vi "AlliGator Phasor Algebra Calculator.vi"(7 "XYGraph in":T7, 8 "error in (no error)":errorcluster, 9 "Phasor Plot Destination":T1, 10 "Phasor Plot Algebra Output":T2 {"1-Exp Lifetime" min=0.0; "Delay" min=0.0}, 11 "Data Value Reference in":refnum<data-value>) -> (0 "error out":errorcluster, 1 "Message":string, 3 "Data Value Reference out":refnum<data-value>)   [LabVIEW 2021, in "AlliGator Phasor Graph.lvlib"]
doc: "Implements user-requested calculations on phsor plots."
uses:
  AlliGator Phasor Graph.lvlib
  AlliGator Internal Variables v2.ctl
  <vilib>/vision/Image Controls.llb/IMAQ Image.ctl
  AlliGator Gate Image Set.ctl
  AlliGator FLI Dataset Type.ctl
  AlliGator Data Series Type.ctl
  AlliGator Dataset Channel.ctl
  AlliGator Gate Arithmetic.ctl
  AlliGator Displayed Image.ctl
  Image/Named ROI Description.ctl
  AlliGator Decay Metadata v3.ctl
  AlliGator Decay Background Subtraction Info.ctl
  AlliGator Baseline Subtraction Method.ctl
  Graphs/XY Graph/XY Graph Plot Shift Parameters.ctl
  Graphs/XY Graph/XY Graph Plot Shift Method.ctl
  AlliGator Decay Extrapolation Parameters.ctl
  Phasor/Calibration Phasor (m, phi).ctl
  Phasor/Phasor Reference Series.ctl
  Phasor/Phasor Calibration Map v2.ctl
  Phasor/Phasor (g, s).ctl
  AlliGator Raw Phasor Plot Data v4.ctl
  Phasor/Phasor Standard Deviation Options.ctl
  AlliGator Phasor Multi-Harmonic Data.ctl
  Phasor/Phasor Harmonic Data.ctl
  AlliGator Decay Fit Options & Parameters v2.ctl
  Fits/IRF(X)PSED/Decay Fit Options v2.ctl
  Fits/Decay Convolution/Decay Model.ctl
  Fits/Residual Type.ctl
  Fits/IRF(X)PSED/Fit Weights Type.ctl
  Fits/Non-linear Fitting Method v2.ctl
  Fits/Fit Calculation Method.ctl
  Fits/Non-linear Fitting Algorithm.ctl
  AlliGator Decay Fit Parameter Constraints 2.ctl
  Fits/IRF(X)PSED/Decay Fit Parameters In List.ctl
  Fits/IRF(X)PSED/MLE Baseline Offset Type.ctl
  AlliGator Decay Preprocessing Parameters.ctl
  Fits/IRF(X)PSED/Decay Fit Parameters & Derived Quantities List.ctl
  Graphs/XY Graph/XY Graph Refnum.ctl
  AlliGator 2-Phasor Plot Multiplication.ctl
  Phasor/Phasor Operation.ctl
  Phasor/Phasor (m, phi).ctl
  Phasor/Phasor Representation.ctl
  AlliGator Phasor Plot Destination.ctl
  Graphs/Plot Point Style.ctl
  Graphs/LabVIEW Plot Interpolation.ctl
  02880097-ea6c-4998-a11e-0251a8662878.vi
  <vilib>/Utility/error.llb/Error Cluster From Error Code.vi
  Math/ix/ix (DBL).vi
  Graphs/XY Graph/XY Graph Add Single Plot with Name.vi
  <vilib>/ErrorRing/Error Ring.xnode
  Graphs/XY Graph/XY Graph Add-Ons.lvlib
  AlliGator Settings.lvlib
  Math/Math.lvlib
  Phasor/Phasor.lvlib
  Graphs/Graphs.lvlib
  Image/Image.lvlib
  AlliGator Decay Preprocessing.lvlib
  AlliGator Files.lvlib
  AlliGator Phasor Plot.lvlib
  AlliGator Source Image.lvlib
  Fits/Fits.lvlib
  AlliGator Decay Fit.lvlib
  AlliGator Decay Fit Parameter Map.lvlib
  AlliGator Internal Variables.lvlib
  AlliGator Dual-Channel Datasets.lvlib
panel:
  # "see the AlliGator License on the block diagram (Ctrl+E or Window:Show Block Diagram)"
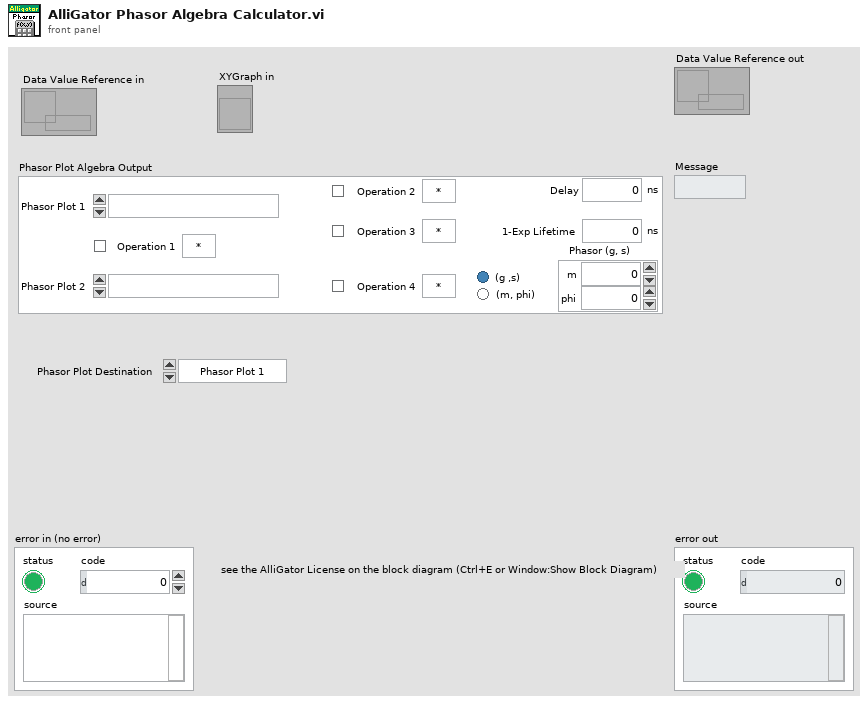
[diagram p1: front panel]
types:
  T1 = typedef "AlliGator Phasor Graph.lvlib/AlliGator Phasor Plot Destination.ctl" = enum32{"Phasor Plot 1", "Phasor Plot 2", "New Phasor Plot"}
  T2 = typedef "AlliGator Phasor Graph.lvlib/AlliGator 2-Phasor Plot Multiplication.ctl" = cluster{"Phasor Plot 1":u16, "Operation 1":T3, "Phasor Plot 2":u16, "Operation 2":T3, "Delay":dbl[unit], "Operation 3":T3, "1-Exp Lifetime":dbl[unit], "Operation 4":T3, "Phasor (g, s)":T4, "Phasor (m, phi)":T5, "Phasor Representation":T6, "Use Operation 1":bool, "Use Operation 2":bool, "Use Operation 3":bool, "Use Operation 4":bool}
  T3 = typedef "Phasor.lvlib/Phasor Operation.ctl" = enum16{"*", "/"}
  T4 = typedef "Phasor.lvlib/Phasor (g, s).ctl" = cluster{"g":dbl, "s":dbl}
  T5 = typedef "Phasor.lvlib/Phasor (m, phi).ctl" = cluster{"m":dbl, "phi":dbl}
  T6 = typedef "Phasor.lvlib/Phasor Representation.ctl" = enum32{"(g, s)", "(m, phi)"}
  T7 = typedef "XY Graph Add-Ons.lvlib/XY Graph Refnum.ctl" = refnum<vi>
  T8 = typedef "Graphs.lvlib/Plot Point Style.ctl" = enum16{"not defined", "None", "Empty Circle", "Filled Circle", "Thick Circle", "Dotted Circle", "Empty Square", "Filled Square", "Thick Square", "Dotted Square", "Small Filled Square", "Dot", "Cross", "Tiny Cross", "Large X", "Small x", "Diamond", "Small Empty Square"}
  T9 = typedef "AlliGator Internal Variables.lvlib/AlliGator Internal Variables v2.ctl" = cluster{"Displayed Image":T10, "White Light Image":T10, "Mask Image":T10, "ROI Mask Image":T10, "Current Dataset Images 1":T11, "Background Dataset Images 1":T11, "Current Dataset Images 2":T11, "Background Dataset Images 2":T11, "Current Dataset Arithmetic Images":T11, "Accumulated Dataset Images 1":T11, "Accumulated Dataset Images 2":T11, "Accumulated Dataset Arithmetic Images":T11, "Phasor Plot Image":T10, "Decay Fit Parameter Map Image":T10, "Single Data Point Path":path, "White Light Image Path":path, "Mask Image Path":path, "Time-Series Folder":path, "[Time-Series Paths]":path[], "Current Dataset":i32, "Single Dataset Type":T12, "Current Folder":string, "AlliGator Data Series Type":T13, "# Datasets":i32, "Dual-Channel Dataset":bool, "Selected Channel Name":string, "Dataset Channel":T14, "Channel Arithmetic":T15, "Dual-Channel Background Dataset":bool, "Background Channel":T14, "Dual-Channel Accumulated Dataset":bool, "Start Time":dbl, "[Time-Series Timestamps]":dbl[], "[Intensity Corrections]":dbl[], "Time Series Script":bool, "Type of Displayed Image":T16, "Gate Image Slide":u16, "# Gates":i32, "ROIs":T17[], "ROI Decay":cluster{"t Array":dbl[], "I Array":dbl[]}, "Valid Decay":bool, "Decay  Metadata":T19, "Reference Decay Plot Name":string, "Reference Decay":cluster{"t Array":dbl[], "I Array":dbl[]}, "Decay Shift Plot":cluster{"Time Stamps":dbl[], "Decay Shifts":dbl[]}, "[Decays Max Values]":sgl[], "[Decays Min Values]":sgl[], "Calibration Phasor":T25, "Calibration Phasor Series":T26, "Phasor Calibration Map":T27, "Calibration Map MD5 Digest":string, "Last Raw Phasor":T4, "Last Calibrated Phasor":T4, "Last Calibrated Phasor SDV":T4, "Phasor Graph:Phasor Plot":cluster{"g Array":dbl[], "s Array":dbl[]}, "Phasor Graph:Phasor SDV Plot":cluster{"g Array":dbl[], "s Array":dbl[]}, "[Phasor Graph:Raw Phasor Plots]":T28[], "Phasor Plot locked to Ref 1":i32, "[Phasor Plot(s) locked to Ref 1]":i32[], "[Phasor Plot(s) locked to Ref 2]":i32[], "[Pixel Phasors]":T4[], "[[Sum Image]]":dbl[][], "[[CSG Phasors]]":csg[][], "[[Valid Pixel?]]":bool[][], "I/m/phi Dataset":cluster{"I/m/phi Dataset?":bool, "Base Frequency":dbl[unit], "Harmonic Orders":u8[]}, "Multi Phasor Plot Data":T30, "Decay Fit Options & Parameters":T32, "Fit Options: Decay Preprocessing Parameters":T43, "Fit Options: Reference Decay":cluster{"t Array":dbl[], "I Array":dbl[]}, "Is Full Image Parameters Map":bool, "Is Single-Pixels Parameters Map":bool, "NLSF Parameters Map X Resolution":i32, "NLSF Parameters Map Y Resolution":i32, "[Single Decay Fit Parameters]":dbl[], "Fit Model":T34, "[[Multiple Decays Fit Parameters]]":dbl[][], "[[Multiple Decays Fit Parameter SDVs]]":dbl[][], "[[IRFs]]":dbl[][], "IRF Array Time Axis":dbl[], "Decay Array Time Axis":dbl[], "[Decay Fit Parameter Names]":T44[], "[[Phasor Ratios]]":dbl[][], "[[Average Lifetimes]]":dbl[][], "Amplitude Weighted Average Lifetime":bool, "[Decay Sum]":dbl[], "[[User-defined Quantities]]":dbl[][], "User-defined Quantity":string}
  T10 = typedef "IMAQ Image.ctl" = refnum<image>
  T11 = typedef "AlliGator Files.lvlib/AlliGator Gate Image Set.ctl" = cluster{"SGL Image Max":T10, "SGL Image Sum":T10, "SGL Gate Images":T10[], "SGL Image Min":T10}
  T12 = typedef "AlliGator Files.lvlib/AlliGator FLI Dataset Type.ctl" = enum16{"HDF5 FLI Dataset", "Gate Image Folder", ".sdt FLI Dataset (Becker & Hickl)", ".ptu FLI Dataset (PicoQuant)", "SS1 FLI Dataset", "SS2 FLI Dataset", "I/m/phi Dataset", ".bin FLI Dataset (PicoQuant Binned)", ".bin FLI Dataset (Piccolo Binned)"}
  T13 = typedef "AlliGator Files.lvlib/AlliGator Data Series Type.ctl" = enum16{"Not a Supported Series", "Gate Images Folder Series", "SwissSPAD 2 Dataset Series", "B&H FLI Dataset Series", "PicoQuant PTU FLI Dataset Series", "PicoQuant BIN FLI Dataset Series", "Piccolo hist BIN FLI Dataset Series", "HDF5 FLI Dataset Series"}
  T14 = typedef "AlliGator Dual-Channel Datasets.lvlib/AlliGator Dataset Channel.ctl" = enum16{"G2", "INT"}
  T15 = typedef "AlliGator Settings.lvlib/AlliGator Gate Arithmetic.ctl" = enum16{"None", "INT-G2", "G2/INT*<INT>", "(1 - G2/INT)*<INT>"}
  T16 = typedef "AlliGator Source Image.lvlib/AlliGator Displayed Image.ctl" = enum16{"Single Gate", "Sum of All Gates", "Max of All Gates", "Min of All Gates", "-", "White Ligth Image", "Mask Image"}
  T17 = typedef "Image.lvlib/Named ROI Description.ctl" = cluster{"ROI Descriptor":T18, "ROI Name":string, "Overlay Color":u32}
  T18 = typedef "ROI Descriptor" = cluster{"Global Rectangle":i32[], "Contours":cluster{"ID":enum32{"External", "Internal"}, "Type":u32, "Coordinates":i32[]}[]}
  T19 = typedef "AlliGator Phasor Graph.lvlib/AlliGator Decay Metadata v3.ctl" = cluster{"ROI Descriptor":T18, "ROI Center":cluster{"X":i32, "Y":i32}, "Decay Background Subtraction Info":T20, "Decay Reverted":bool, "Decay Smoothened":bool, "Decay Straightened":bool, "Fitted Tau (Decay Straightening)":dbl, "Decay Shift Parameters":T22, "Decay Shifted":bool, "Decay Extrapolated":bool, "Decay Extrapolation Parameters":T24, "Decay Normalized":bool, "Fold Decay":bool, "# Folds":u32}
  T20 = typedef "AlliGator Decay Analysis.lvlib/AlliGator Decay Preprocessing.lvlib/AlliGator Decay Background Subtraction Info.ctl" = cluster{"Laser Period":dbl[unit], "Gate Duration":dbl[unit], "Baseline Subtraction Method":T21, "Background Definition Range":cluster{"Min Gate":dbl[unit], "Max Gate":dbl[unit]}, "Total Intensity w/o Bkgd Subtraction":dbl, "Bkgd-subtracted Intensity (exp)":dbl, "# Data Points":i32, "Background/Gate":dbl, "Fitted Lifetime":dbl[unit], "Bkgd-subtracted Intensity (theo)":dbl}
  T21 = typedef "AlliGator Decay Analysis.lvlib/AlliGator Decay Preprocessing.lvlib/AlliGator Baseline Subtraction Method.ctl" = enum16{"Mean", "Min", "Square Gated Single-Exponential", "File", "Constant"}
  T22 = typedef "XY Graph Add-Ons.lvlib/XY Graph Plot Shift Parameters.ctl" = cluster{"Type":T23, "Shift":dbl[unit], "Threshold":dbl, "Rotate":bool}
  T23 = typedef "XY Graph Add-Ons.lvlib/XY Graph Plot Shift Method.ctl" = enum16{"Default", "CFD", "Threshold", "Cross-Correlation"}
  T24 = typedef "AlliGator Decay Analysis.lvlib/AlliGator Decay Preprocessing.lvlib/AlliGator Decay Extrapolation Parameters.ctl" = cluster{"Additional Points":u32, "Head Fraction":dbl, "Fitted Tau":dbl, "Use Periodicity":bool, "Use Cursors":bool, "Tail Fraction":dbl}
  T25 = typedef "Phasor.lvlib/Calibration Phasor (m, phi).ctl" = cluster{"m":dbl, "phi":dbl, "Phasor Frequency":dbl[unit], "Reference Lifetime":dbl[unit]}
  T26 = typedef "Phasor.lvlib/Phasor Reference Series.ctl" = cluster{"m Array":dbl[], "phi Array":dbl[], "Phasor Frequency":dbl[unit], "Calibration Lifetime":dbl[unit]}
  T27 = typedef "Phasor.lvlib/Phasor Calibration Map v2.ctl" = cluster{"Phasor Frequency":dbl[unit], "Calibration Lifetime":dbl[unit], "ROI Centers":cluster{"X":i32, "Y":i32}[], "ROI Descriptors":T18[], "Map Resolution X":i32, "Map Resolution Y":i32, "z Array":cdb[]}
  T28 = typedef "AlliGator Phasor Graph.lvlib/AlliGator Raw Phasor Plot Data v4.ctl" = cluster{"Phasor Plot Name":string, "Raw Phasor Plot":T4[], "Phasor Frequency":dbl[unit], "[Decay Metadata]":T19[], "Raw Phasor Plot SDV":T4[], "Phasor SDV Options":T29, "[Calibration Phasor]":T25[]}
  T29 = typedef "Phasor.lvlib/Phasor Standard Deviation Options.ctl" = cluster{"Compute Estimated SDV":bool, "# Replicas":u32, "Use Estimated Average Phasor":bool}
  T30 = typedef "AlliGator Phasor Plot.lvlib/AlliGator Phasor Multi-Harmonic Data.ctl" = cluster{"Base Frequency":dbl[unit], "# Harmonics":u8, "Harmonic Orders":u8[], "Phasor Plot Settings Checksum":u64, "Phasor Harmonic Data Array":T31[]}
  T31 = typedef "Phasor.lvlib/Phasor Harmonic Data.ctl" = cluster{"Phasor Harmonic Name":string, "Phasor Plot Settings Checksum":u64, "Phasor Frequency":dbl[unit], "Base Frequency":dbl[unit], "Harmonic Order":u8, "Phasor Plot Parameters":string, "Phasor Array [[CSG]]":csg[][], "Dataset File Path":path}
  T32 = typedef "AlliGator Decay Fit Parameter Map.lvlib/AlliGator Decay Fit Options & Parameters v2.ctl" = cluster{"SYNC Period":dbl[unit], "Fit Options":T33, "Fit Parameter Constraints":T40[], "MLE Baseline Offset":dbl, "MLE Baseline Offset Type":T42}
  T33 = typedef "Fits.lvlib/Decay Fit Options v2.ctl" = cluster{"Show Fit Residuals":bool, "Fit Model":T34, "Residual Type":T35, "Max Decay Percentile":dbl, "Min Decay Percentile":dbl, "Show Full Decay":bool, "Weights":T36, "Fitting Method":T37, "Compute Parameter Uncertainties":bool, "Periodic Boundaries":bool, "Model Calculation":T38, "Period":dbl[unit], "Termination Criteria":cluster{"Max Iterations":i32, "Max Function Calls":i32, "Max Time":dbl[unit], "Function Tolerance":dbl, "Parameter Tolerance":dbl, "Gradient Tolerance":dbl, "Min Lambda":dbl, "Max Lambda":dbl, "Initial Tick Count":u32}, "Offset Resolution":dbl[unit], "Use Local IRF":bool, "Fitting Algorithm":T39}
  T34 = typedef "Fits.lvlib/Decay Model.ctl" = enum16{"1-Exponential", "2-Exponentials"}
  T35 = typedef "Fits.lvlib/Residual Type.ctl" = enum16{"Standard", "Normalized", "Reduced"}
  T36 = typedef "Fits.lvlib/Fit Weights Type.ctl" = enum16{"Unweighted", "1/Variance", "Best of All"}
  T37 = typedef "Fits.lvlib/Non-linear Fitting Method v2.ctl" = enum16{"Least Square", "Least Absolute Residual", "Bisquare", "MLE", "-", "Best of All"}
  T38 = typedef "Fits.lvlib/Fit Calculation Method.ctl" = enum16{"Simulation", "Convolution", "Integration"}
  T39 = typedef "Fits.lvlib/Non-linear Fitting Algorithm.ctl" = enum16{"Levenberg-Marquardt", "Trust-Region Dogleg"}
  T40 = typedef "AlliGator Decay Analysis.lvlib/AlliGator Decay Fit.lvlib/AlliGator Decay Fit Parameter Constraints 2.ctl" = cluster{"Fit Parameter":T41, "Min Value":dbl, "Max Value":dbl, "Global":bool, "Used":bool}
  T41 = typedef "Fits.lvlib/Decay Fit Parameters In List.ctl" = enum16{"Offset", "Baseline", "A_1", "tau_1", "A_2", "tau_2"}
  T42 = typedef "Fits.lvlib/MLE Baseline Offset Type.ctl" = enum32{"Absolute", "Percentage"}
  T43 = typedef "AlliGator Decay Analysis.lvlib/AlliGator Decay Preprocessing.lvlib/AlliGator Decay Preprocessing Parameters.ctl" = cluster{"Background Subtraction":bool, "Straighten Decay":bool, "Reverse Gates":bool, "1-Normalized Decay":bool, "Smoothen Decay":bool, "Smoothing Parameter":dbl, "Shift Decay":bool, "Decay Shift Parameters":T22, "Extrapolate Decay":bool, "Additional Points":u32, "Head Fraction":dbl, "Pixel-Normalize Decay":bool, "Use Periodicity":bool, "Use Cursors":bool, "Tail Fraction":dbl, "Use Decay Pre-Processing":bool, "Fold Decay":bool, "# Folds":u32, "[0-1]-Normalized Decay":bool}
  T44 = typedef "Fits.lvlib/Decay Fit Parameters & Derived Quantities List.ctl" = enum16{"Offset", "Baseline", "A_1", "tau_1", "A_2", "tau_2", "<tau>_a", "f1_a", "f2_a", "<tau>_i", "f1_i", "f2_i", "-", "R^2", "Chi^2"}
  T45 = typedef "XY Graph Add-Ons.lvlib/XY Plot Data.ctl" = cluster{"X Array":dbl[], "Y Array":dbl[]}
  T46 = typedef "Graphs.lvlib/LabVIEW Plot Interpolation.ctl" = u8
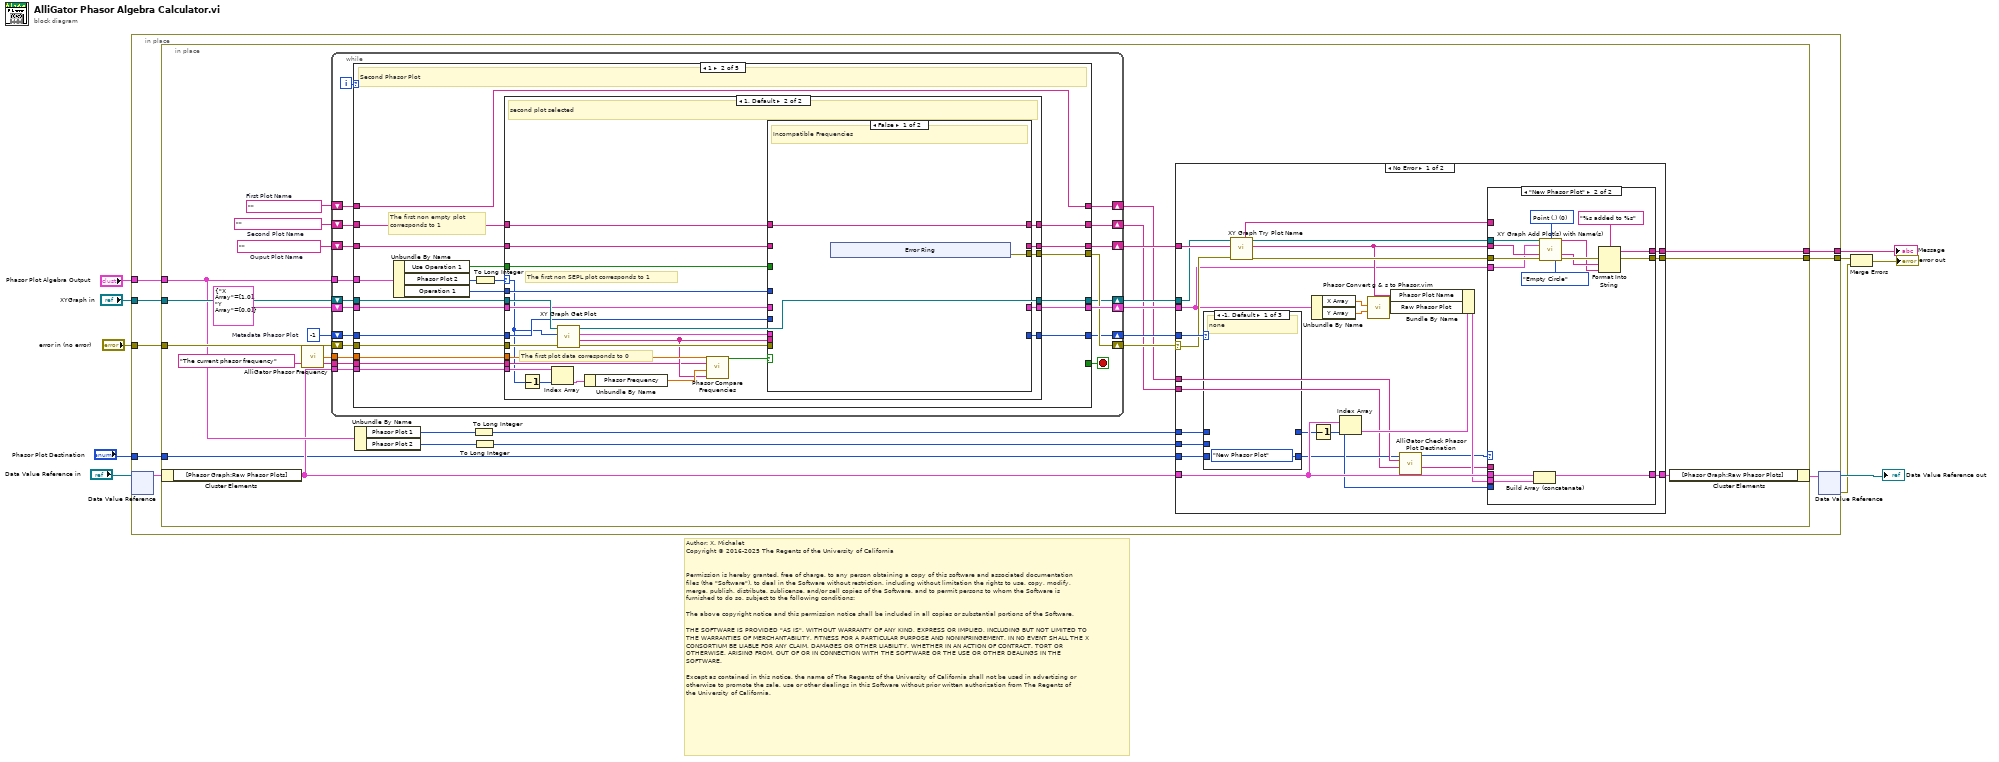
[diagram p0: block diagram]
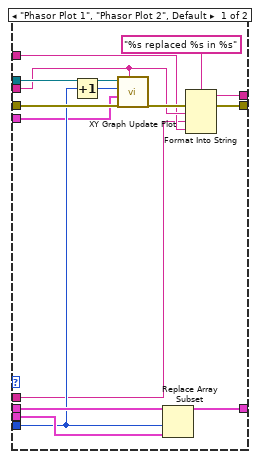
[diagram p2: hidden frame]
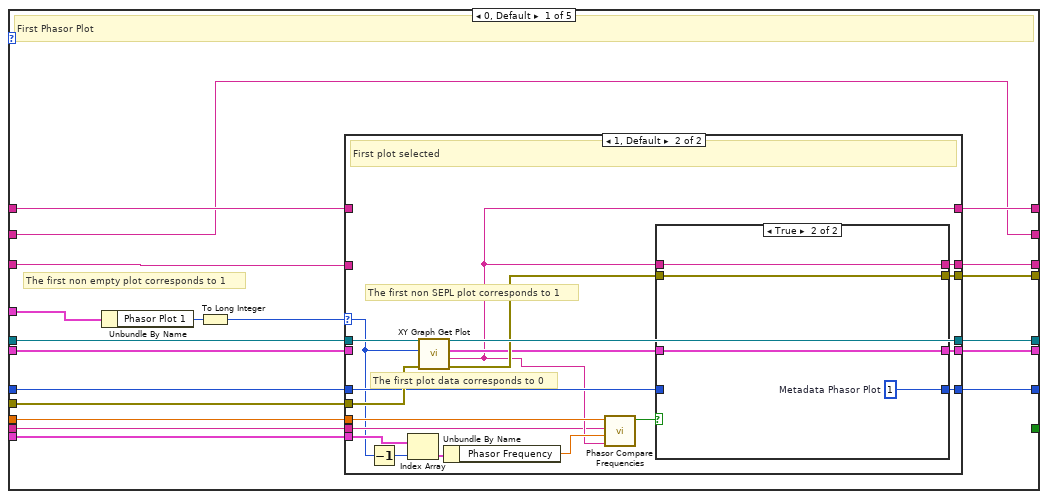
[diagram p6: hidden frame]
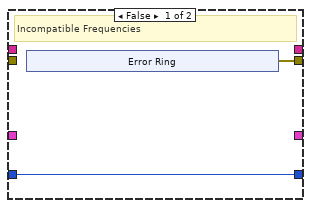
[diagram p8: hidden frame]
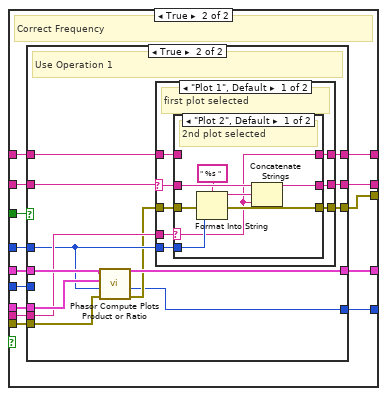
[diagram p10: hidden frame]
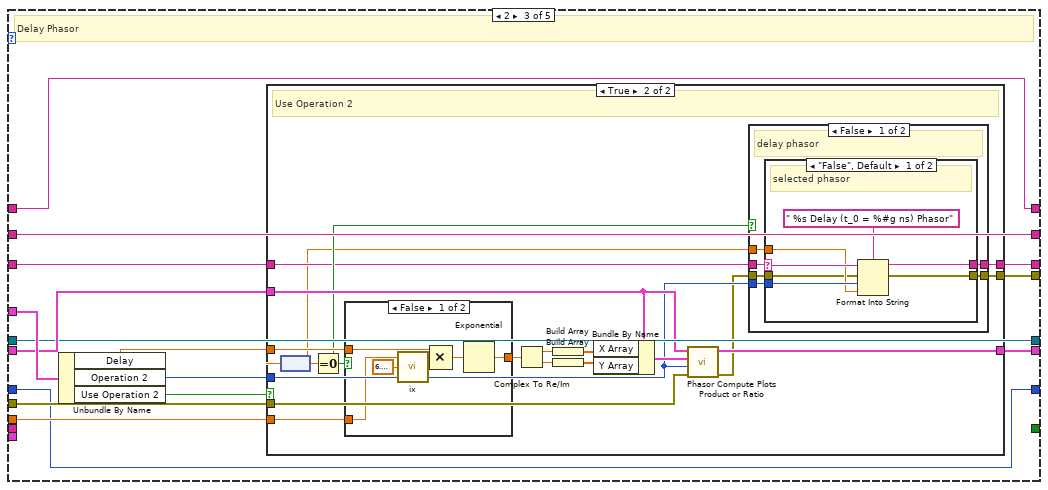
[diagram p14: hidden frame]
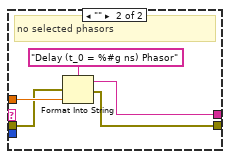
[diagram p16: hidden frame]
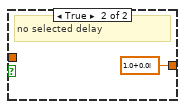
[diagram p18: hidden frame]
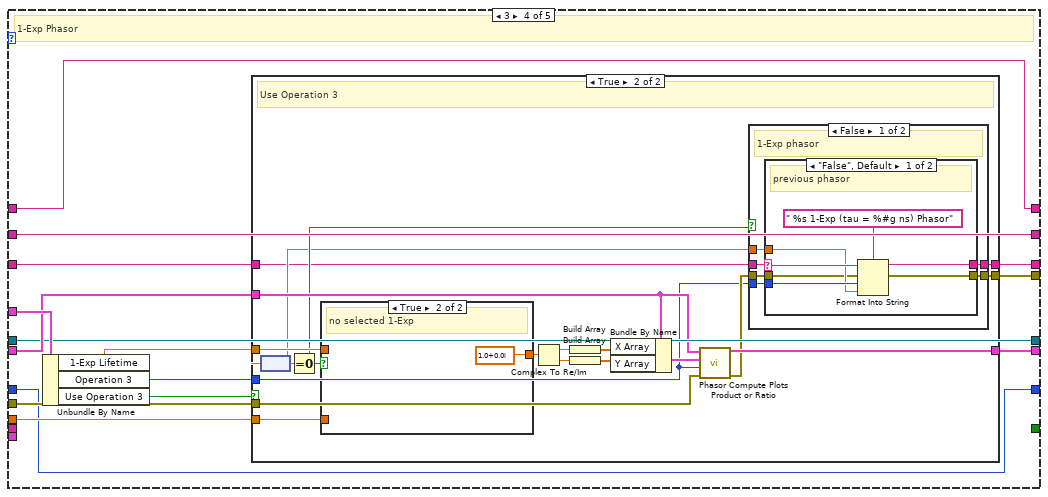
[diagram p19: hidden frame]
diagram:
  # "Author: X. Michalet\nCopyright © 2016-2025 The Regents of the University of California\n \n\nPermission is hereby granted, free of charge, to any person obtaining a copy of this software and associated documentation files (the \"Software\"), to deal in the Software without restriction, including without limitation the rights to use, copy, modify, merge, publish, distribute, sublicense, and/or sell copies of the Software, and to permit persons to whom the Software is furnished to do so, subject to the following conditions:\n\nThe above copyright notice and this permission notice shall be included in all copies or substantial portions of the Software.\n\nTHE SOFTWARE IS PROVIDED \"AS IS\", WITHOUT WARRANTY OF ANY KIND, EXPRESS OR IMPLIED, INCLUDING BUT NOT LIMITED TO THE WARRANTIES OF MERCHANTABILITY, FITNESS FOR A PARTICULAR PURPOSE AND NONINFRINGEMENT. IN NO EVENT SHALL THE X CONSORTIUM BE LIABLE FOR ANY CLAIM, DAMAGES OR OTHER LIABILITY, WHETHER IN AN ACTION OF CONTRACT, TORT OR OTHERWISE, ARISING FROM, OUT OF OR IN CONNECTION WITH THE SOFTWARE OR THE USE OR OTHER DEALINGS IN THE SOFTWARE.\n\nExcept as contained in this notice, the name of The Regents of the University of California shall not be used in advertising or otherwise to promote the sale, use or other dealings in this Software without prior written authorization from The Regents of the University of California."
  n1 = in-place {
    in-place-border: "Phasor Plot Algebra Output" -> [w18]
    in-place-border: "XYGraph in" -> [w16]
    in-place-border: "error in (no error)" -> [w15]
    in-place-border: [w13] -> w4
    in-place-border: [w12] -> w5
    in-place-border: "Phasor Plot Destination" -> [w11]
    n2 = in-place-dvr #1("Data Value Reference in") -> (w17:T9)  [unwired: 1 out]
    n3 = in-place {
      in-place-border: w18 -> [w40]
      in-place-border: w16 -> [w44]
      in-place-border: w15 -> [w43]
      in-place-border: [w26] -> w13
      in-place-border: [w25] -> w12
      in-place-border: w11 -> [w20]
      w23 = ""  # Second Plot Name
      w24 = ""  # First Plot Name
      w36 = -1  # Metadata Phasor Plot
      w39 = ""  # Ouput Plot Name
      n4 = in-place-cluster #2(w17) -> ("[Phasor Graph:Raw Phasor Plots]"=w29:T28[])
      n5 = call "AlliGator Phasor Frequency.vi"() -> ("Phasor Frequency"=w42:dbl[unit])
      n6 = while {
        tunnel: w40 -> [w129]
        shift-right: [w119] -> w38
        shift-left: w43 -> [w127]
        shift-right: [w126] -> w30
        shift-left: cluster{"X Array":dbl[], "Y Array":dbl[]} {"X Array"=[1.0], "Y Array"=[0.0]} ("Plot Data") -> [w124]
        tunnel: w42 -> [w123]
        shift-right: [w120] -> w27
        shift-left: w39 -> [w121]
        shift-right: [w118] -> w28
        shift-left: w44 -> [w128]
        shift-right: [w116] -> w35
        shift-left: w36 -> [w117]
        tunnel: w29 -> [w115]
        shift-right: [w114] -> w22
        shift-left: w24 -> [w113]
        shift-right: [w111] -> w21
        shift-left: w23 -> [w112]
        tunnel: "The current phasor frequency" ("Phasor Frequency 1 Name") -> [w110]
        i -> [w125]
        stop <- w122 stop-if-true
        n7 = case shown="1" w125 {
          tunnel: w129 -> [w148 w204 w309 w372 w439]
          tunnel: w128 -> [w146 w202 w299 w362 w427]
          tunnel: w127 -> [w145 w201 w304 w367 w435]
          tunnel: [w144 w197 w306 w368 w436] -> w126
          tunnel: w124 -> [w142 w199 w305 w369 w437]
          tunnel: w123 -> [w134 w189 w307 w370 _]
          tunnel: [_ _ _ _ TRUE] -> w122
          tunnel: w121 -> [w141 w196 w303 w366 w434]
          tunnel: [w140 w195 w302 w364 w432] -> w120
          tunnel: [w139 w194 w300 w365 w433] -> w119
          tunnel: [w138 w193 w299 w362 w427] -> w118
          tunnel: w117 -> [w137 w192 w296 w359 w429]
          tunnel: [w136 w191 w296 w359 w429] -> w116
          tunnel: w115 -> [w135 w190 _ _ _]
          tunnel: [w133 w185 w297 w360 w430] -> w114
          tunnel: w113 -> [w132 w185 w297 w360 w430]
          tunnel: w112 -> [w131 w188 w298 w361 w426]
          tunnel: [w131 w187 w298 w361 w426] -> w111
          tunnel: w110 -> [w130 w184 _ _ _]
          frame 0, Default {
            # "The first non empty plot corresponds to 1"
            # "First Phasor Plot"
            n8 = Unbundle By Name(w148) -> ("Phasor Plot 1"=w147:u16)
            n9 = To Long Integer(number=w147) -> (32bit integer=w143:i32)
            n10 = case shown="1, Default" w143 {
              selector: w143 -> [_ w155]
              tunnel: w146 -> [w151 w173]
              tunnel: w145 -> [w154 w172]
              tunnel: [w153 w161] -> w144
              tunnel: [w154 w162] -> w139
              tunnel: w142 -> [w153 _]
              tunnel: w141 -> [w152 _]
              tunnel: [w152 w163] -> w140
              tunnel: [w151 w171] -> w138
              tunnel: w137 -> [w150 w160]
              tunnel: [w150 w170] -> w136
              tunnel: w135 -> [_ w169]
              tunnel: w134 -> [_ w167]
              tunnel: [w149 w157] -> w133
              tunnel: w132 -> [w149 _]
              tunnel: w130 -> [_ w156]
              frame 0 {
                # "no selected plot"
              }
              frame 1, Default {
                # "The first plot data corresponds to 0"
                # "The first non SEPL plot corresponds to 1"
                # "First plot selected"
                n11 = Decrement(x=w155) -> (x-1=w159:i32)
                n12 = Index Array(array=w169, index=w159) -> (element=w168:T28)
                n13 = call "XY Graph Get Plot.vi"("error in (no error)"=w172, "Plot Index (-1: last)"=w155, "XYGraph in"=w173) -> ("error out"=w165:errorcluster, "Plot Name"=w157:string, "Plot Data"=w164:T45, "XYGraph out"=w171:T7)  [unwired: 4 in, 1 out]
                n14 = Unbundle By Name(w168) -> ("Phasor Frequency"=w158:dbl[unit])
                n15 = call "Phasor Compare Frequencies.vi"("Phasor Frequency 2 Name"=w157, "Phasor Frequency 2"=w158, "Phasor Frequency 1 Name"=w156, "Phasor Frequency 1"=w167) -> ("Accept?"=w166:bool)  [unwired: 7 in]
                n16 = case shown="True" w166 {
                  tunnel: [w174 w183] -> w170
                  tunnel: w157 -> [_ w182]
                  tunnel: w165 -> [_ w181]
                  tunnel: w164 -> [_ w180]
                  tunnel: [_ w182] -> w163
                  tunnel: [w175 w181] -> w162
                  tunnel: [_ w180] -> w161
                  tunnel: w160 -> [w174 _]
                  frame False {
                    # "Incompatible Frequencies"
                    n17 = xnode "Error Ring"() -> ("error out"=w175:errorcluster)
                  }
                  frame True {
                    w183 = 1  # Metadata Phasor Plot
                  }
                }
              }
            }
          }
          frame 1 {
            # "The first non empty plot corresponds to 1"
            # "Second Phasor Plot"
            n18 = Unbundle By Name(w204) -> ("Use Operation 1"=w186:bool, "Phasor Plot 2"=w203:u16, "Operation 1"=w198:T3)
            n19 = To Long Integer(number=w203) -> (32bit integer=w200:i32)
            n20 = case shown="1, Default" w200 {
              selector: w200 -> [_ w211]
              tunnel: w202 -> [w207 w235]
              tunnel: w201 -> [w208 w234]
              tunnel: w199 -> [w210 w231]
              tunnel: w198 -> [_ w227]
              tunnel: [w210 w233] -> w197
              tunnel: w196 -> [w209 w229]
              tunnel: [w209 w228] -> w195
              tunnel: [w208 w226] -> w194
              tunnel: [w207 w225] -> w193
              tunnel: w192 -> [w206 w217]
              tunnel: [w206 w224] -> w191
              tunnel: w190 -> [_ w223]
              tunnel: w189 -> [_ w216]
              tunnel: w188 -> [w205 w221]
              tunnel: [w205 w220] -> w187
              tunnel: w186 -> [_ w218]
              tunnel: w184 -> [_ w213]
              frame 0 {
                # "no selected plot"
              }
              frame 1, Default {
                # "The first plot data corresponds to 0"
                # "The first non SEPL plot corresponds to 1"
                # "second plot selected"
                n21 = Decrement(x=w211) -> (x-1=w219:i32)
                n22 = Index Array(array=w223, index=w219) -> (element=w222:T28)
                n23 = call "XY Graph Get Plot.vi"("error in (no error)"=w234, "Plot Index (-1: last)"=w211, "XYGraph in"=w235) -> ("error out"=w232:errorcluster, "Plot Name"=w214:string, "Plot Data"=w230:T45, "XYGraph out"=w225:T7)  [unwired: 4 in, 1 out]
                n24 = Unbundle By Name(w222) -> ("Phasor Frequency"=w215:dbl[unit])
                n25 = call "Phasor Compare Frequencies.vi"("Phasor Frequency 2 Name"=w214, "Phasor Frequency 2"=w215, "Phasor Frequency 1 Name"=w213, "Phasor Frequency 1"=w216) -> ("Accept?"=w212:bool)  [unwired: 7 in]
                n26 = case shown="False" w212 {
                  tunnel: [_ w255] -> w233
                  tunnel: w232 -> [_ w254]
                  tunnel: w231 -> [_ w253]
                  tunnel: w230 -> [_ w252]
                  tunnel: w229 -> [_ w251]
                  tunnel: w214 -> [_ w250]
                  tunnel: [_ w249] -> w228
                  tunnel: w227 -> [_ w248]
                  tunnel: [w237 w247] -> w226
                  tunnel: [_ w246] -> w224
                  tunnel: w221 -> [w236 w245]
                  tunnel: [w236 w244] -> w220
                  tunnel: w218 -> [_ w243]
                  tunnel: w217 -> [_ w242]
                  frame False {
                    # "Incompatible Frequencies"
                    n27 = xnode "Error Ring"() -> ("error out"=w237:errorcluster)
                  }
                  frame True {
                    # "Correct Frequency"
                    n28 = case shown="True" w243 {
                      tunnel: [w257 w273] -> w255
                      tunnel: w254 -> [w258 w272]
                      tunnel: w253 -> [w257 w271]
                      tunnel: w252 -> [_ w270]
                      tunnel: w251 -> [w259 w269]
                      tunnel: w250 -> [_ w268]
                      tunnel: [w259 w267] -> w249
                      tunnel: w248 -> [_ w266]
                      tunnel: [w258 w264] -> w247
                      tunnel: [w256 w263] -> w246
                      tunnel: w245 -> [w260 w262]
                      tunnel: [w260 w261] -> w244
                      tunnel: w242 -> [w256 _]
                      frame False {
                        # "Don't use Operation 1"
                      }
                      frame True {
                        # "Use Operation 1"
                        n29 = call "Phasor Compute Plots Product or Ratio.vi"("error in (no error)"=w272, "Operation"=w266, "Phasor Plot 2"=w270, "Phasor Plot 1"=w271) -> ("error out"=w265:errorcluster, "Metadata Phasor Plot"=w263:i32, "Phasor Plot out"=w273:cluster{"X Array":dbl[], "Y Array":dbl[]})  [unwired: 5 in]
                        n30 = case shown="\"Plot 1\", Default" w269 {
                          selector: w269 -> [w280 _]
                          tunnel: w268 -> [w281 w293]
                          tunnel: [w279 w293] -> w267
                          tunnel: w266 -> [w278 _]
                          tunnel: w265 -> [w277 w294]
                          tunnel: [w276 w294] -> w264
                          tunnel: w262 -> [w275 _]
                          tunnel: [w274 w293] -> w261
                          frame "Plot 1", Default {
                            # "first plot selected"
                            n31 = case shown="\"Plot 2\", Default" w281 {
                              selector: w281 -> [w282 _]
                              tunnel: w280 -> [w289 w292]
                              tunnel: [w286 w292] -> w279
                              tunnel: w278 -> [w287 _]
                              tunnel: w277 -> [w284 w291]
                              tunnel: [w283 w291] -> w276
                              tunnel: w275 -> [_ w290]
                              tunnel: [w282 w290] -> w274
                              frame "Plot 2", Default {
                                # "2nd plot selected"
                                n32 = Format Into String(format string=" %s ", error in=w284, w287) -> (resulting string=w288:string, error out=w283:errorcluster)  [unwired: 1 in]
                                n33 = Concatenate Strings(w289, w288, w282) -> (w286:string)
                              }
                              frame "" {
                                # "no second plot selected"
                              }
                            }
                          }
                          frame "" {
                            # "no first plot selected"
                          }
                        }
                      }
                    }
                  }
                }
              }
            }
          }
          frame 2 {
            # "Delay Phasor"
            n34 = Unbundle By Name(w309) -> ("Delay"=w308:dbl[unit], "Operation 2"=w301:T3, "Use Operation 2"=w295:bool)
            n35 = case shown="True" w295 {
              tunnel: w308 -> [_ w330]
              tunnel: w307 -> [_ w329]
              tunnel: [w310 w322] -> w306
              tunnel: w305 -> [w310 w321]
              tunnel: w304 -> [w311 w320]
              tunnel: w303 -> [w312 w318]
              tunnel: [w312 w317] -> w302
              tunnel: w301 -> [_ w316]
              tunnel: [w311 w313] -> w300
              frame False {
                # "Don't use Operation 2"
              }
              frame True {
                # "Use Operation 2"
                n36 = node(w330) -> (w315:dbl)
                n37 = Equal To 0?(x=w315) -> (x = 0?=w319:bool)
                n38 = case shown="False" w319 {
                  tunnel: w330 -> [w356 _]
                  tunnel: w329 -> [w355 _]
                  tunnel: [w351 cdb 1.0+0.0i] -> w328
                  frame False {
                    n39 = call-poly "ix.vi"("x (1)"=6.283185307179586) -> ("i.(x)"=w354:cdb)
                    n40 = Compound Arithmetic op=MULTIPLY(w356, w355, w354) -> (w352:cdb)
                    n41 = Exponential(1:w352) -> (0:w351:cdb)
                  }
                  frame True {
                    # "no selected delay"
                  }
                }
                n42 = Complex To Re/Im(x + iy=w328) -> (x=w327:dbl, y=w326:dbl)
                n43 = Build Array(w327) -> (w325:dbl[])
                n44 = Build Array(w326) -> (w324:dbl[])
                n45 = Bundle By Name(cluster=w321, "X Array"=w325, "Y Array"=w324) -> (w323:T45)
                n46 = call "Phasor Compute Plots Product or Ratio.vi"("error in (no error)"=w320, "Operation"=w316, "Phasor Plot 2"=w323, "Phasor Plot 1"=w321) -> ("error out"=w314:errorcluster, "Phasor Plot out"=w322:cluster{"X Array":dbl[], "Y Array":dbl[]})  [unwired: 5 in, 1 out]
                n47 = case shown="False" w319 {
                  tunnel: w318 -> [w336 w350]
                  tunnel: [w333 w350] -> w317
                  tunnel: w316 -> [w334 _]
                  tunnel: w315 -> [w335 _]
                  tunnel: w314 -> [w332 w349]
                  tunnel: [w331 w349] -> w313
                  frame False {
                    # "delay phasor"
                    n48 = case shown="\"False\", Default" w336 {
                      selector: w336 -> [w343 _]
                      tunnel: w335 -> [w341 w348]
                      tunnel: w334 -> [w342 _]
                      tunnel: [w339 w346] -> w333
                      tunnel: w332 -> [w338 w345]
                      tunnel: [w337 w344] -> w331
                      frame "False", Default {
                        # "selected phasor"
                        n49 = Format Into String(format string=" %s Delay (t_0 = %#g ns) Phasor", initial string=w343, error in=w338, w342, w341) -> (resulting string=w339:string, error out=w337:errorcluster)
                      }
                      frame "" {
                        # "no selected phasors"
                        n50 = Format Into String(format string="Delay (t_0 = %#g ns) Phasor", error in=w345, w348) -> (resulting string=w346:string, error out=w344:errorcluster)  [unwired: 1 in]
                      }
                    }
                  }
                  frame True {
                    # "no delay"
                  }
                }
              }
            }
          }
          frame 3 {
            # "1-Exp Phasor"
            n51 = Unbundle By Name(w372) -> ("1-Exp Lifetime"=w371:dbl[unit], "Operation 3"=w363:T3, "Use Operation 3"=w358:bool)
            n52 = case shown="True" w358 {
              tunnel: w371 -> [_ w393]
              tunnel: w370 -> [_ w392]
              tunnel: w369 -> [w373 w385]
              tunnel: [w373 w384] -> w368
              tunnel: w367 -> [w374 w383]
              tunnel: w366 -> [w375 w380]
              tunnel: [w374 w378] -> w365
              tunnel: [w375 w377] -> w364
              tunnel: w363 -> [_ w376]
              frame False {
                # "Don't use Operation 3"
              }
              frame True {
                # "Use Operation 3"
                n53 = node(w393) -> (w381:dbl)
                n54 = Equal To 0?(x=w381) -> (x = 0?=w382:bool)
                n55 = case shown="True" w382 {
                  tunnel: w393 -> [w421 _]
                  tunnel: w392 -> [w420 _]
                  tunnel: [w414 cdb 1.0+0.0i] -> w387
                  frame False {
                    n56 = call-poly "ix.vi"("x (1)"=6.283185307179586) -> ("i.(x)"=w419:cdb)
                    n57 = Compound Arithmetic op=MULTIPLY(w421, w420, w419) -> (w417:cdb)
                    n58 = Decrement(x=w417) -> (x-1=w416:cdb)
                    n59 = Negate(x=w416) -> (-x=w415:cdb)
                    n60 = Reciprocal(x=w415) -> (1/x=w414:cdb)
                  }
                  frame True {
                    # "no selected 1-Exp"
                  }
                }
                n61 = Complex To Re/Im(x + iy=w387) -> (x=w391:dbl, y=w390:dbl)
                n62 = Build Array(w391) -> (w389:dbl[])
                n63 = Build Array(w390) -> (w388:dbl[])
                n64 = Bundle By Name(cluster=w385, "X Array"=w389, "Y Array"=w388) -> (w386:T45)
                n65 = call "Phasor Compute Plots Product or Ratio.vi"("error in (no error)"=w383, "Operation"=w376, "Phasor Plot 2"=w386, "Phasor Plot 1"=w385) -> ("error out"=w379:errorcluster, "Phasor Plot out"=w384:cluster{"X Array":dbl[], "Y Array":dbl[]})  [unwired: 5 in, 1 out]
                n66 = case shown="False" w382 {
                  tunnel: w380 -> [w399 w413]
                  tunnel: [w396 w413] -> w377
                  tunnel: w376 -> [w397 _]
                  tunnel: w381 -> [w398 _]
                  tunnel: w379 -> [w395 w412]
                  tunnel: [w394 w412] -> w378
                  frame False {
                    # "1-Exp phasor"
                    n67 = case shown="\"False\", Default" w399 {
                      selector: w399 -> [w406 _]
                      tunnel: w398 -> [w404 w411]
                      tunnel: w397 -> [w405 _]
                      tunnel: [w402 w409] -> w396
                      tunnel: w395 -> [w401 w408]
                      tunnel: [w400 w407] -> w394
                      frame "False", Default {
                        # "previous phasor"
                        n68 = Format Into String(format string=" %s 1-Exp (tau = %#g ns) Phasor", initial string=w406, error in=w401, w405, w404) -> (resulting string=w402:string, error out=w400:errorcluster)
                      }
                      frame "" {
                        # "no previous phasors"
                        n69 = Format Into String(format string="1-Exp (tau = %#g ns) Phasor", error in=w408, w411) -> (resulting string=w409:string, error out=w407:errorcluster)  [unwired: 1 in]
                      }
                    }
                  }
                  frame True {
                    # "no 1-Exp"
                  }
                }
              }
            }
          }
          frame 4 {
            # "User-entered Phasor"
            n70 = Unbundle By Name(w439) -> ("Phasor Representation"=w425:T6, "Phasor (g, s)"=w424:T4, "Phasor (m, phi)"=w423:T5, "Operation 4"=w431:T3, "Use Operation 4"=w428:bool)
            n71 = case shown="True" w428 {
              tunnel: w437 -> [w440 w457]
              tunnel: [w440 w456] -> w436
              tunnel: w435 -> [w441 w445]
              tunnel: w434 -> [w442 w455]
              tunnel: [w441 w453] -> w433
              tunnel: [w442 w452] -> w432
              tunnel: w431 -> [_ w451]
              tunnel: w425 -> [_ w450]
              tunnel: w424 -> [_ w449]
              tunnel: w423 -> [_ w446]
              frame False {
                # "Don't use Operation 4"
              }
              frame True {
                # "Use Operation 4"
                n72 = case shown="\"(g, s)\", Default" w450 {
                  tunnel: w449 -> [w476 _]
                  tunnel: [w472 w486] -> w448
                  tunnel: [w471 w485] -> w447
                  tunnel: w446 -> [_ w483]
                  tunnel: w445 -> [w475 w480]
                  tunnel: [w474 w479] -> w444
                  tunnel: [w473 w478] -> w443
                  frame "(g, s)", Default {
                    n73 = Unbundle By Name(w476) -> ("g"=w472:dbl, "s"=w471:dbl)
                    n74 = Format Into String(format string="%#g + i %#g", error in=w475, w472, w471) -> (resulting string=w473:string, error out=w474:errorcluster)  [unwired: 1 in]
                  }
                  frame "(m, phi)" {
                    # "no selected 1-Exp"
                    n75 = Unbundle By Name(w483) -> ("m"=w482:dbl, "phi"=w481:dbl)
                    n76 = Polar To Complex(1:w481, 2:w482) -> (0:w484:cdb)
                    n77 = Format Into String(format string="%#g e^i %#g", error in=w480, w482, w481) -> (resulting string=w478:string, error out=w479:errorcluster)  [unwired: 1 in]
                    n78 = Complex To Re/Im(x + iy=w484) -> (x=w486:dbl, y=w485:dbl)
                  }
                }
                n79 = Build Array(w448) -> (w460:dbl[])
                n80 = Build Array(w447) -> (w459:dbl[])
                n81 = Bundle By Name(cluster=w457, "X Array"=w460, "Y Array"=w459) -> (w458:T45)
                n82 = call "Phasor Compute Plots Product or Ratio.vi"("error in (no error)"=w444, "Operation"=w451, "Phasor Plot 2"=w458, "Phasor Plot 1"=w457) -> ("error out"=w454:errorcluster, "Phasor Plot out"=w456:cluster{"X Array":dbl[], "Y Array":dbl[]})  [unwired: 5 in, 1 out]
                n83 = case shown="\"\"" w455 {
                  selector: w455 -> [w467 _]
                  tunnel: w451 -> [w466 _]
                  tunnel: [w464 w469] -> w452
                  tunnel: w454 -> [w463 w468]
                  tunnel: [w462 w468] -> w453
                  tunnel: w443 -> [w461 w469]
                  frame "False", Default {
                    # "previous phasor"
                    n84 = Format Into String(format string=" %s %s", initial string=w467, error in=w463, w466, w461) -> (resulting string=w464:string, error out=w462:errorcluster)
                  }
                  frame "" {
                    # "no previous phasors"
                  }
                }
              }
            }
          }
        }
      }
      n85 = Unbundle By Name(w40) -> ("Phasor Plot 1"=w34:u16, "Phasor Plot 2"=w33:u16)
      n86 = To Long Integer(number=w34) -> (32bit integer=w32:i32)
      n87 = To Long Integer(number=w33) -> (32bit integer=w31:i32)
      n88 = case shown="No Error" w38 {
        selector: w38 -> [w64 w108]
        tunnel: w29 -> [w72 w109]
        tunnel: [w68 w109] -> w37
        tunnel: w20 -> [w50 _]
        tunnel: w35 -> [w71 _]
        tunnel: w32 -> [w70 _]
        tunnel: w31 -> [w69 _]
        tunnel: w30 -> [w53 _]
        tunnel: w28 -> [w62 _]
        tunnel: w27 -> [w63 _]
        tunnel: [w59 w108] -> w26
        tunnel: [w58 _] -> w25
        tunnel: w22 -> [w48 _]
        tunnel: w21 -> [w46 _]
        frame No Error {
          n89 = case shown="-1, Default" w71 {
            tunnel: [_ w105 w107] -> w67
            tunnel: w70 -> [_ w105 _]
            tunnel: w69 -> [_ _ w107]
            tunnel: w50 -> [_ w104 w106]
            tunnel: [AlliGator_Phasor_Plot_Destination."New Phasor Plot" ("Phasor Plot Destination") w104 w106] -> w47
            frame -1, Default {
              # "none"
            }
            frame 1 {
              # "first plot"
            }
            frame 2 {
              # "second plot"
            }
          }
          n90 = call "XY Graph Try Plot Name.vi"("Error In"=w64, "Plot Name in"=w63, "XY Graph Refnum"=w62) -> ("Error Out"=w61:errorcluster, "Plot Name out"=w54:string, "XY Graph Refnum"=w60:T7, "Graph Caption (or Label)"=w52:string)  [unwired: 5 in]
          n91 = Unbundle By Name(w53) -> ("X Array"=w56:dbl[], "Y Array"=w55:dbl[])
          n92 = Decrement(x=w67) -> (x-1=w57:i32)
          n93 = Index Array(array=w72, index=w57) -> (element=w51:T28)
          n94 = call "Phasor Convert g & s to Phasor.vim"("s"=w55, "g"=w56) -> ("Phasor Array"=w65:T4[])  [unwired: 8 in]
          n95 = Bundle By Name(cluster=w51, "Phasor Plot Name"=w54, "Raw Phasor Plot"=w65) -> (w66:T28)
          n96 = call "AlliGator Check Phasor Plot Destination.vi"("Second Plot Name"=w46, "First Plot Name"=w48, "Phasor Plot Destination in"=w47) -> ("Destination Plot Name"=w45:string, "Phasor Plot Destination out"=w49:T1)  [unwired: 7 in]
          n97 = case shown="\"New Phasor Plot\"" w49 {
            tunnel: w72 -> [w87 w102]
            tunnel: [w86 w101] -> w68
            tunnel: w66 -> [w85 w100]
            tunnel: w61 -> [w83 w97]
            tunnel: w60 -> [w84 w96]
            tunnel: [w78 w94] -> w59
            tunnel: [w73 w90] -> w58
            tunnel: w57 -> [w81 _]
            tunnel: w54 -> [w77 w89]
            tunnel: w53 -> [w79 w88]
            tunnel: w52 -> [w76 _]
            tunnel: w45 -> [w75 _]
            frame "Phasor Plot 1", "Phasor Plot 2", Default {
              n98 = Increment(x=w81) -> (x+1=w80:i32)
              n99 = call "XY Graph Update Plot.vi"("New Plot Name (Default: unchanged)"=w77, "Error In"=w83, "Plot"=w79, "Plot Idx"=w80, "XY Graph refnum"=w84) -> ("Error Out"=w82:errorcluster)  [unwired: 6 in]
              n100 = Replace Array Subset(array=w87, new element=w85, index=w81) -> (w86:T28[])
              n101 = Format Into String(format string="%s replaced %s in %s", error in=w82, w77, w75, w76) -> (resulting string=w73:string, error out=w78:errorcluster)  [unwired: 1 in]
            }
            frame "New Phasor Plot" {
              w99 = T46 0 items=["Point (.)", "Stepwise Right (--.)", "Line + Point (\\. /)", "Stepwise Left (.--)", "Stepwise Centered (-.-)", "Stepwise Vertical (|.|)", "Line (-)", "Use Previous Plot's Style"] ("Plot Interpolation (Previous Plot's Style)")
              n102 = Build Array (concatenate)(w102, w100) -> (w101:T28[])
              n103 = call-poly "XY Graph Add Plot(s) with Name(s).vi"("XYGraph Ref in"=w96, "Plot Interpolation (Previous Plot's Style)"=w99, "Plot"=w88, "Plot Name (\"Plot\")"=w89, "error in (no error)"=w97, "Point Style (Dot)"=Plot_Point_Style."Empty Circle") -> ("XY Graph Caption (or Label)"=w92:string, "Plot Name"=w93:string, "error out"=w95:errorcluster)  [unwired: 6 in, 1 out]
              n104 = Format Into String(format string="%s added to %s", error in=w95, w93, w92) -> (resulting string=w90:string, error out=w94:errorcluster)  [unwired: 1 in]
            }
          }
        }
        frame Error {
        }
      }
      n105 = in-place-cluster #2("[Phasor Graph:Raw Phasor Plots]"=w37) -> (w14:T9)
    }
    n106 = in-place-dvr #1(w14) -> (→"Data Value Reference out":refnum<data-value>, w2:errorcluster)
  }
  "Message" <- w5
  n107 = Merge Errors(w4, w2) -> (→"error out":errorcluster)
